vi "gate_controller.vi"() -> ()   [LabVIEW 2010]
panel:
  in  "Command":T1(ring)=enum."Read Voltage"
  in  "Numerical Argument":i32
  out "Response":string
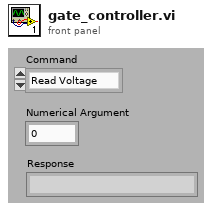
[diagram p1: front panel]
types:
  T1 = enum16{"Set Voltage", "Read Voltage", "Read Setpoint", "Read Current", "Output On", "Output Off"}
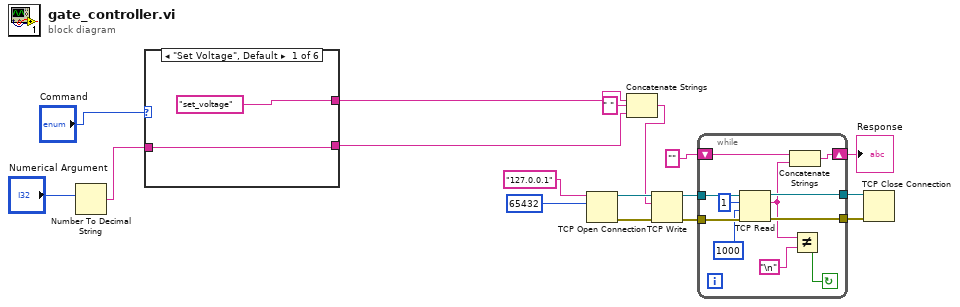
[diagram p0: block diagram]
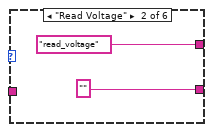
[diagram p2: hidden frame]
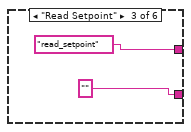
[diagram p3: hidden frame]
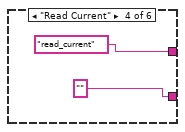
[diagram p4: hidden frame]
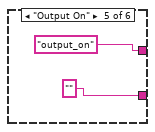
[diagram p5: hidden frame]
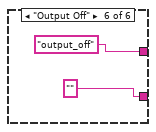
[diagram p6: hidden frame]
diagram:
  n1 = Number To Decimal String(number="Numerical Argument") -> (decimal integer string=w1:string)  [unwired: 1 in]
  n2 = case shown="\"Set Voltage\", Default" "Command" {
    tunnel: ["set_voltage" ("data in") "read_voltage" ("data in") "read_setpoint" ("data in") "read_current" ("data in") "output_on" ("data in") "output_off" ("data in")] -> w6
    tunnel: [w18 "" ("string") "" ("string") "" ("string") "" ("string") "" ("string")] -> w2
    tunnel: w1 -> [w18 _ _ _ _ _]
    frame "Set Voltage", Default {
    }
    frame "Read Voltage" {
    }
    frame "Read Setpoint" {
    }
    frame "Read Current" {
    }
    frame "Output On" {
    }
    frame "Output Off" {
    }
  }
  n3 = TCP Open Connection(address="127.0.0.1", remote port or service name=u16 65432) -> (connection ID=w15:refnum<k5>, error out=w14:errorcluster)  [unwired: 3 in]
  n4 = Concatenate Strings(w6, " " ("string"), w2) -> (w7:string)
  n5 = TCP Write(connection ID=w15, data in=w7, error in (no error)=w14) -> (connection ID out=w12:refnum<k5>, error out=w13:errorcluster)  [unwired: 1 in, 1 out]
  n6 = while {
    tunnel: w13 -> [w40]
    tunnel: w12 -> [w39]
    tunnel: [w38] -> w11
    tunnel: [w37] -> w10
    shift-right: [w33] -> w8
    shift-left: "" ("string") -> [w34]
    stop <- w32 continue-if-true
    n7 = TCP Read(connection ID=w39, bytes to read=1, error in (no error)=w40, 9:1000 ("timeout ms (25000)")) -> (connection ID out=w37:refnum<k5>, data out=w31:string, error out=w38:errorcluster)  [unwired: 1 in]
    n8 = Concatenate Strings(w34, w31) -> (w33:string)
    n9 = Not Equal?(x=w31, y="\n") -> (x != y?=w32:bool)
  }
  "Response" <- w8
  n10 = TCP Close Connection(connection ID=w10, error in (no error)=w11) -> ()  [unwired: 1 in, 2 out]
